vi "Read Current and Voltage Measurement and Step Source.vi"(8 "error in (no error)":errorcluster, 9 "Source Value (0.1)":dbl=0.1, 10 "Source Measure Unit Channel (0: Channel A)":i32(ring) items=["Channel A", "Channel B"], 11 "VISA resource name":refnum<visa-resource-name>) -> (0 "error out":errorcluster, 1 "Voltage (V)":dbl, 2 "Current (A)":dbl, 3 "VISA resource name out":refnum<visa-resource-name>)   [LabVIEW 2020, in "Keithley 2600 Series.lvlib"]
doc: "Returns the measured current and voltage before stepping the source."
uses:
  <instrlib>/Keithley 2600 Series/Keithley 2600 Series.lvlib
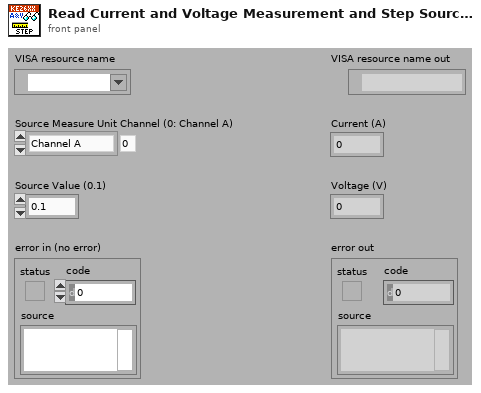
[diagram p1: front panel]
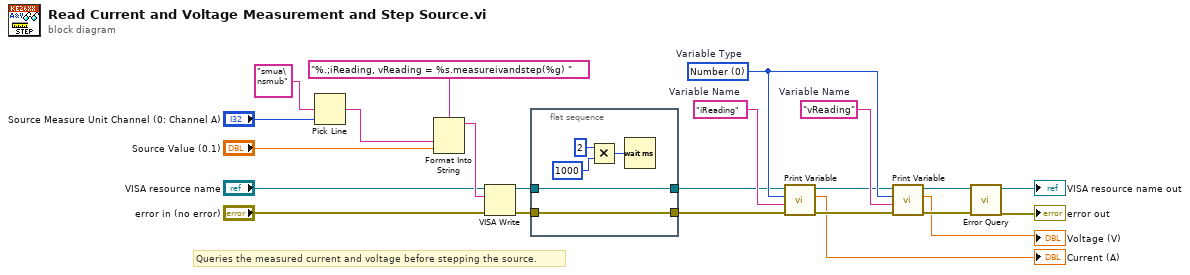
[diagram p0: block diagram]
diagram:
  w10 = "vReading"  # Variable Name
  w11 = "iReading"  # Variable Name
  w9 = 0 items=["Number", "Message"]  # Variable Type
  # "Queries the measured current and voltage before stepping the source."
  n1 = Pick Line(multi-line string="smua\nsmub", line index="Source Measure Unit Channel (0: Channel A)") -> (output string=w14:string)  [unwired: 1 in]
  n2 = Format Into String(format string="%.;iReading, vReading = %s.measureivandstep(%g) ", w14, "Source Value (0.1)") -> (resulting string=w21:string)  [unwired: 2 in, 1 out]
  n3 = VISA Write(VISA resource name="VISA resource name", write buffer=w21, error in (no error)="error in (no error)") -> (VISA resource name out=w13:refnum<visa-resource-name>, error out=w12:errorcluster)  [unwired: 1 out]
  n4 = flat-sequence {
    tunnel: w13 -> [w28]
    tunnel: w12 -> [w27]
    tunnel: [w28] -> w8
    tunnel: [w27] -> w7
    frame #0 {
      n5 = Multiply(x=2, y=1000) -> (x*y=w25:i32)
      n6 = Wait (ms)(milliseconds to wait=w25) -> ()  [unwired: 1 out]
    }
  }
  n7 = call <instrlib>:"Print Variable.vi"("error in (no error)"=w7, "Variable Name"=w11, "Variable Type (0: Number)"=w9, "VISA resource name"=w8) -> ("error out"=w5:errorcluster, "Number"=→"Current (A)":dbl, "VISA resource name out"=w6:refnum<visa-resource-name>)  [unwired: 4 in, 1 out]
  n8 = call <instrlib>:"Print Variable.vi"("error in (no error)"=w5, "Variable Name"=w10, "Variable Type (0: Number)"=w9, "VISA resource name"=w6) -> ("error out"=w3:errorcluster, "Number"=→"Voltage (V)":dbl, "VISA resource name out"=w4:refnum<visa-resource-name>)  [unwired: 4 in, 1 out]
  n9 = call <instrlib>:"Error Query.vi"("error in (no error)"=w3, "VISA resource name"=w4) -> ("error out"=→"error out":errorcluster, "VISA resource name out"=→"VISA resource name out":refnum<visa-resource-name>)  [unwired: 6 in, 2 out]
